vi "Standalone Pump.vi"() -> ()   [LabVIEW 2014]
uses:
  Pump.Simulated class/Pump.Simulated.lvclass
  Pump class/Pump.lvclass/Pump.ctl
  Pump class/Pump State - cluster.ctl
  <vilib>/JKI/JKI SMO/SMO/SMO.lvclass
  Pump class/Pump.lvclass
panel:
  out "Pump State":T1(graph)
  in  "Speed Command":dbl
  in  "Apply Setpoint":bool
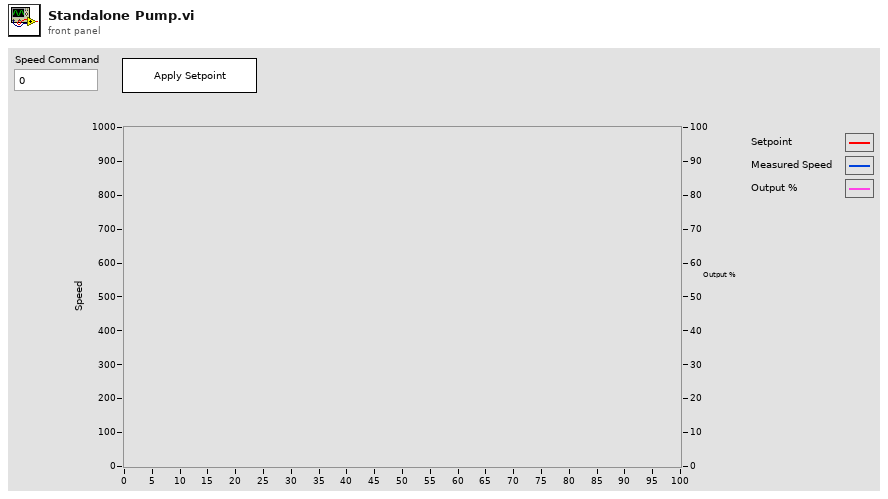
[diagram p1: front panel]
types:
  T1 = typedef "Pump.lvclass/Pump State - cluster.ctl" = cluster{"Pump Setpoint":dbl, "Pump Speed":dbl, "Output %":dbl}
  T2 = typedef "SMO.lvclass/Public Events.ctl" = cluster{"Error":refnum<user-event>, "State":refnum<user-event>, "Reserve State":refnum<user-event>}
  T3 = typedef "SMO.lvclass/SMOState --Enum.ctl" = enum16{"unknown", "Created", "Started", "Stopped"}
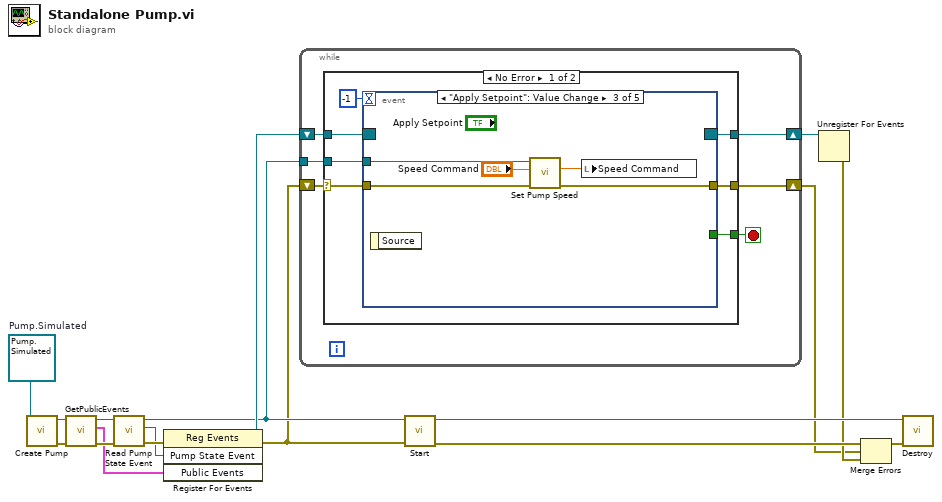
[diagram p0: block diagram]
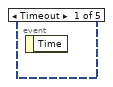
[diagram p2: hidden frame]
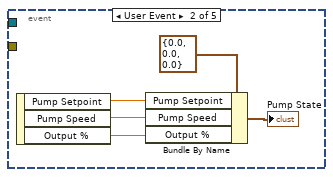
[diagram p3: hidden frame]
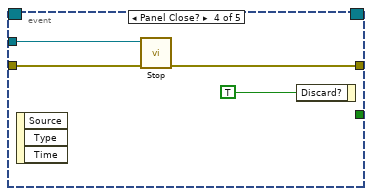
[diagram p4: hidden frame]
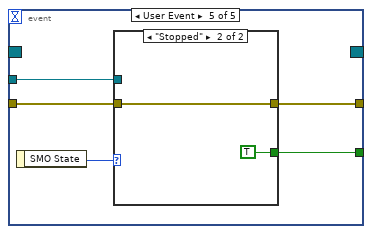
[diagram p5: hidden frame]
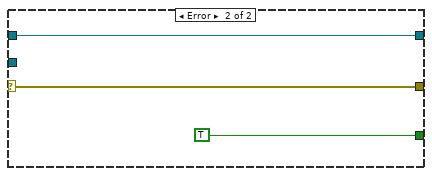
[diagram p7: hidden frame]
diagram:
  w1 = refnum<class "Pump.Simulated.lvclass"> refnum  # Pump.Simulated
  n1 = call "Create Pump.vi"("Pump in"=w1) -> ("error out"=w13:errorcluster, "Pump out"=w15:refnum<class "Pump.Simulated.lvclass">)  [unwired: 8 in, 1 out]
  n2 = call <vilib>:"GetPublicEvents.vi"("error in (no error)"=w13, "SMO"=w15) -> ("error out"=w12:errorcluster, "Public Events"=w11:T2, "SMO out"=w14:refnum<class "Pump.Simulated.lvclass">)  [unwired: 7 in]
  n3 = call "Read Pump State Event.vi"("error in (no error)"=w12, "Pump in"=w14) -> ("error out"=w17:errorcluster, "Pump State Event"=w16:refnum<user-event>, "Pump out"=w8:refnum<class "Pump.Simulated.lvclass">)  [unwired: 7 in]
  n4 = register-events(error in=w17, w16, w11) -> (reference out=w9:refnum<event-registration>, error out=w2:errorcluster)  [unwired: 1 in]
  n5 = while {
    shift-right: [w22] -> w10
    shift-left: w9 -> [w23]
    shift-right: [w19] -> w3
    shift-left: w2 -> [w20]
    tunnel: w8 -> [w18]
    stop <- w21 stop-if-true
    n6 = case shown="No Error" w20 {
      selector: w20 -> [w25 w53]
      tunnel: w23 -> [w29 w55]
      tunnel: [w28 w55] -> w22
      tunnel: [w27 TRUE] -> w21
      tunnel: [w24 w53] -> w19
      tunnel: w18 -> [w26 _]
      frame No Error {
        n7 = event shown="[2] \"Apply Setpoint\": Value Change" {
          selector: w29 -> [_ _ _ _ _]
          dyn-events: [_ _ _ _ _] -> w28
          timeout: -1 -> [_ _ _ _ _]
          tunnel: [_ _ _ _ w49] -> w27
          tunnel: w26 -> [_ _ w38 w44 w47]
          tunnel: w25 -> [_ _ w40 w43 w45]
          tunnel: [_ _ w39 w42 w46] -> w24
          event Timeout {
            n8 = event-data() -> ()  [unwired: 1 in, 1 out]
          }
          event User Event {
            n9 = event-data() -> ("Pump Setpoint"=w34:dbl, "Pump Speed"=w32:dbl, "Output %"=w31:dbl)  [unwired: 1 in]
            n10 = Bundle By Name(cluster=T1 {"Pump Setpoint"=0.0, "Pump Speed"=0.0, "Output %"=0.0} ("Pump State"), "Pump Setpoint"=w34, "Pump Speed"=w32, "Output %"=w31) -> (→"Pump State":T1)
          }
          event "Apply Setpoint": Value Change {
            n11 = event-data() -> ()  [unwired: 1 in, 1 out]
            n12 = call "Set Pump Speed.vi"("error in (no error)"=w40, "Speed Command"="Speed Command", "Pump in"=w38) -> ("error out"=w39:errorcluster, "Pump Setpoint"=w36:dbl)  [unwired: 5 in, 2 out]
            n13 = local write "Speed Command"(w36) -> ()
          }
          event Panel Close? {
            n14 = event-data() -> ()  [unwired: 1 in, 3 out]
            n15 = call <vilib>:"Stop.vi"("error in (no error)"=w43, "SMO"=w44) -> ("error out"=w42:errorcluster)  [unwired: 8 in, 1 out]
            n16 = event-data("Discard?"=TRUE) -> ()  [unwired: 1 in, 1 out]
          }
          event User Event {
            n17 = event-data() -> ("SMO State"=w48:T3)  [unwired: 1 in]
            n18 = case shown="\"Stopped\"" w48 {
              tunnel: [_ TRUE] -> w49
              tunnel: w47 -> [_ _]
              tunnel: [w50 w51] -> w46
              tunnel: w45 -> [w50 w51]
              frame Default {
              }
              frame "Stopped" {
              }
            }
          }
        }
      }
      frame Error {
      }
    }
  }
  n19 = call <vilib>:"Start.vi"("error in (no error)"=w2, "SMO"=w8) -> ("error out"=w7:errorcluster, "SMO out"=w5:refnum<class "Pump.Simulated.lvclass">)  [unwired: 8 in]
  n20 = Unregister For Events(event registration refnum=w10) -> (error out=w4:errorcluster)  [unwired: 1 in]
  n21 = Merge Errors(w7, w3, w4) -> (w6:errorcluster)
  n22 = call <vilib>:"Destroy.vi"("error in (no error)"=w6, "SMO"=w5) -> ()  [unwired: 9 in, 1 out]
